vi "Test MeaSplit.vi"() -> ()   [LabVIEW 2019, in "XCP_DaqDtoId.lvlib" / "DAQList.lvclass"]
uses:
  DAQList.lvclass
  DAQList.lvclass/DAQList.ctl
  XnetRead/SubVI_MergeData2.vi
  <vilib>/xnet/xnet.llb/XNET String To IO Name (Database Filepath).vi
  TypeDef/Global.vi
  <vilib>/ECUMC/ECUMC.llb/MC Get Property.vi
  <vilib>/ECUMC/ECUMC.llb/MC Get Prop Meas Data Type.vi
  <vilib>/xnet/xnet.llb/XNET Database Close (Database).vi
  <resource>/objmgr/xnet.rc
panel:
  in  "DAQList Databse File Path":path=path "C:/LVLibrary/XNET/XCP_DaqDTOID/XCP_DaqDTOId/DAQList/Test/DAQLists_Short.xml"
  out "Merged Data":dbl[](array[numeric]) format="%#.2f"
  in  "Data Part 2":dbl[](array[numeric])=[6.06e-39]
  in  "Data Part 1":dbl[](array[numeric])=[2.242e-44]
  out "Error Out":errorcluster
  # "0x10"
  # "0xD1 0xFC 0x41"
  # "0x10 0xD1 0xFC 0x41"
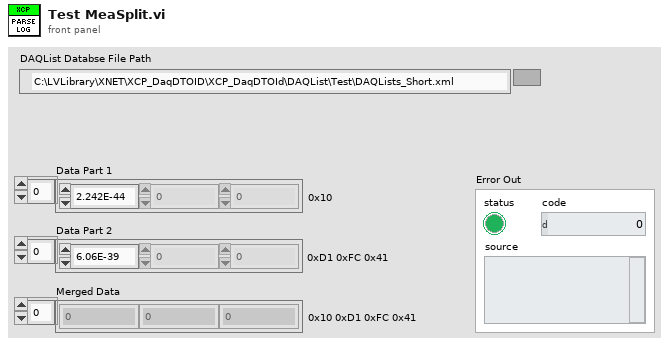
[diagram p1: front panel]
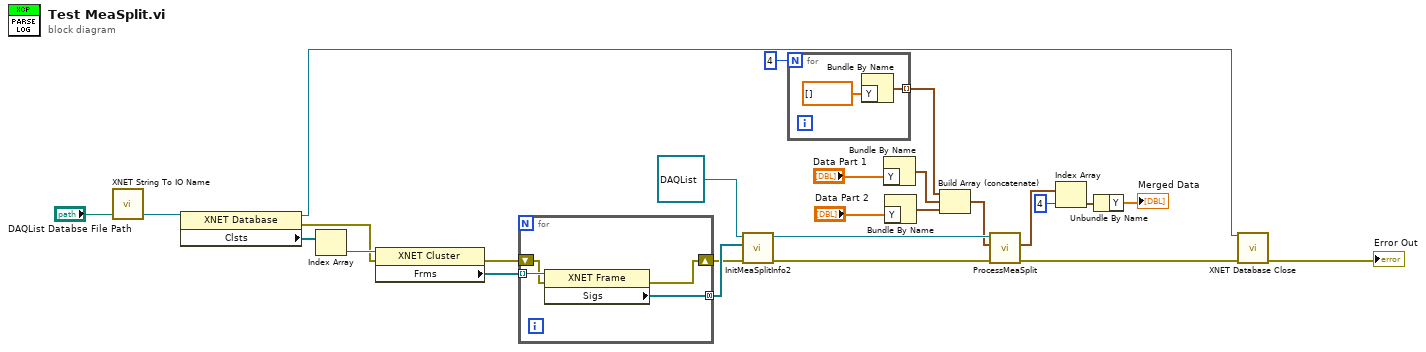
[diagram p0: block diagram]
diagram:
  n1 = call-poly <vilib>:"XNET String To IO Name.vi"("filepath"="DAQList Databse File Path") -> ("XNET Database"=w22:refnum<k21>)  [unwired: 4 out]
  n2 = property class="XNET Database"(reference=w22) -> (reference out=w17:refnum<k21>, error out=w19:errorcluster, "Clsts"=w21:refnum<k21>[])  [unwired: 1 in]
  n3 = Index Array(array=w21) -> (element=w20:refnum<k21>)  [unwired: 1 in]
  n4 = property class="XNET Cluster"(reference=w20, error in=w19) -> (error out=w14:errorcluster, "Frms"=w16:refnum<k21>[])  [unwired: 1 out]
  n5 = for {
    tunnel: w16 -> [w30] mode=indexing
    tunnel: [w29] -> w15 mode=concatenating
    shift-right: [w27] -> w13
    shift-left: w14 -> [w28]
    n6 = property class="XNET Frame"(reference=w30, error in=w28) -> (error out=w27:errorcluster, "Sigs"=w29:refnum<k21>[])  [unwired: 1 out]
  }
  n7 = call "InitMeaSplitInfo2.vi"("error in (no error)"=w13, "Measurement Signals"=w15, "DAQList in"=refnum<class "DAQList.lvclass"> refnum) -> ("error out"=w25:errorcluster, "DAQList out"=w26:refnum<class "DAQList.lvclass">)  [unwired: 7 in]
  n8 = for {
    N: 4 -> [_]
    tunnel: [w31] -> w2 mode=indexing
    n9 = Bundle By Name("Y"=dbl[] []) -> (w31:waveform(dbl))  [unwired: 1 in]
  }
  n10 = Bundle By Name("Y"="Data Part 1") -> (w9:waveform(dbl))  [unwired: 1 in]
  n11 = Bundle By Name("Y"="Data Part 2") -> (w8:waveform(dbl))  [unwired: 1 in]
  n12 = Build Array (concatenate)(w2, w9, w8) -> (w7:waveform(dbl)[])
  n13 = call "ProcessMeaSplit.vi"("error in (no error)"=w25, "Data In"=w7, "DAQList in"=w26) -> ("error out"=w24:errorcluster, "Data Out"=w6:waveform(dbl)[])  [unwired: 6 in, 1 out]
  n14 = Index Array(array=w6, index=4) -> (element=w5:waveform(dbl))
  n15 = Unbundle By Name(w5) -> ("Y"=→"Merged Data":dbl[])
  n16 = call-poly <vilib>:"XNET Database Close.vi"("database in"=w17, "error in (no error)"=w24) -> ("error out"=→"Error Out":errorcluster)  [unwired: 13 in]
